vi "TDT-AODO-Engine.vi"(0 "Config":T1, 2 "Action":T3, 5 "AO":dbl[][](array[numeric]), 7 "DO":bool[][](array[boolean]), 11 "error in (no error)":errorcluster) -> (6 "next buffer":i32, 8 "Space Available":dbl, 15 "error out":errorcluster)   [LabVIEW 2020]
uses:
  Typedefs/TDT-AODO-Action.ctl
  Typedefs/TDT-AODO-Config.ctl
  Typedefs/TDT-AODO-Output Spec.ctl
  TDT-Globals.vi
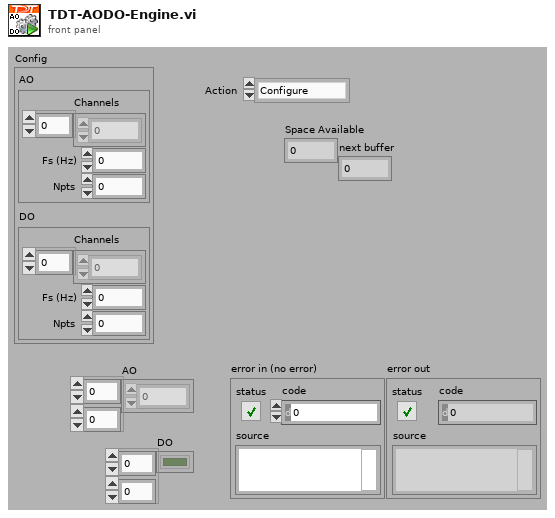
[diagram p1: front panel]
types:
  T1 = typedef "TDT-AODO-Config.ctl" = cluster{"AO":T2, "DO":T2}
  T2 = typedef "TDT-AODO-Output Spec.ctl" = cluster{"Channels":i32[], "Fs (Hz)":dbl, "Npts":i32}
  T3 = typedef "TDT-AODO-Action.ctl" = enum16{"Configure", "Initialize", "Start", "Stop", "Write", "Clean up", "Space available"}
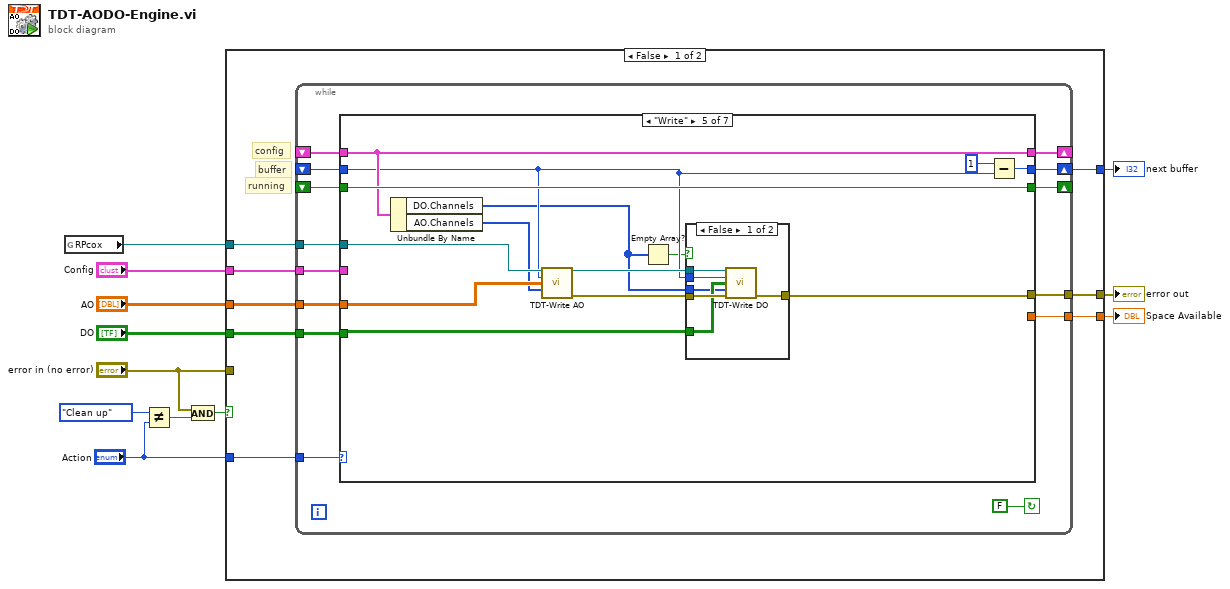
[diagram p0: block diagram]
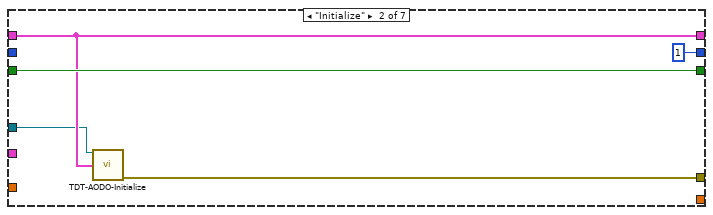
[diagram p3: hidden frame]
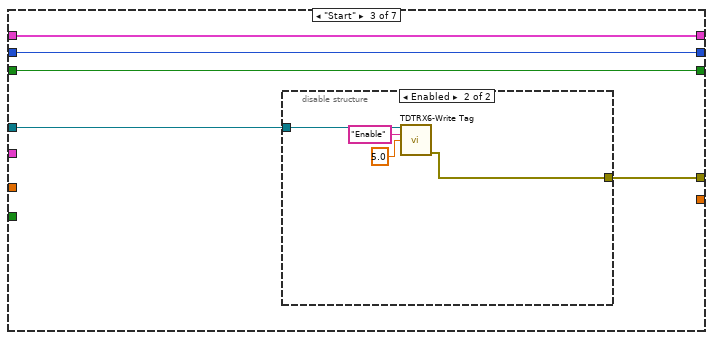
[diagram p4: hidden frame]
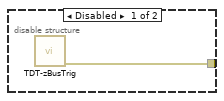
[diagram p5: hidden frame]
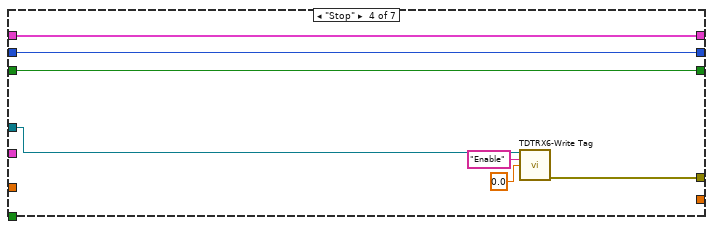
[diagram p6: hidden frame]
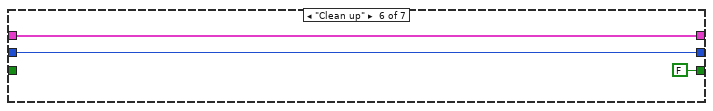
[diagram p8: hidden frame]
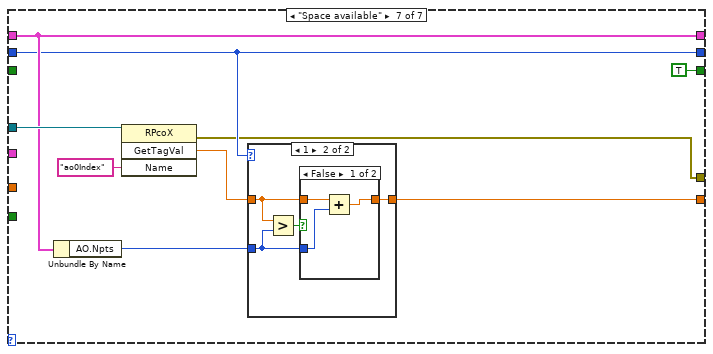
[diagram p9: hidden frame]
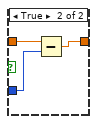
[diagram p11: hidden frame]
diagram:
  n1 = global read "TDT-Globals.vi" "RPcox"() -> (w2:refnum<k7>)
  n2 = Not Equal?(x=TDT-AODO-Action."Clean up", y="Action") -> (x != y?=w6:bool)
  n3 = And(x="error in (no error)", y=w6) -> (x .and. y?=w7:bool)
  n4 = case shown="False" w7 {
    tunnel: "Action" -> [w20 _]
    tunnel: [w19 w104] -> w12
    tunnel: "Config" -> [w18 _]
    tunnel: "AO" -> [w17 _]
    tunnel: "error in (no error)" -> [_ w104]
    tunnel: "DO" -> [w16 _]
    tunnel: [w15 _] -> w3
    tunnel: w2 -> [w14 _]
    tunnel: [w13 _] -> w1
    frame False {
      # "running"
      # "config"
      # "buffer"
      n5 = while {
        shift-right: [w28] -> w13
        shift-left: _ -> [w33]
        tunnel: [w32] -> w19
        tunnel: w18 -> [w30]
        shift-right: [w31] -> _
        shift-left: _ -> [w29]
        tunnel: w17 -> [w27]
        tunnel: w16 -> [w26]
        tunnel: w20 -> [w34]
        tunnel: [w24] -> w15
        shift-right: [w23] -> _
        shift-left: _ -> [w22]
        tunnel: w14 -> [w21]
        stop <- FALSE continue-if-true
        n6 = case shown="\"Write\"" w34 {
          tunnel: [_ w41 w44 w54 w71 _ w84] -> w32
          tunnel: w33 -> [w36 _ w46 w58 w62 w83 w88]
          tunnel: [w37 w40 w47 w59 w68 w82 w90] -> w31
          tunnel: w30 -> [w37 _ _ _ _ _ _]
          tunnel: w29 -> [_ w40 w47 w59 w68 w82 w90]
          tunnel: [w36 1 w46 w58 w64 w83 w88] -> w28
          tunnel: w27 -> [_ _ _ _ w69 _ _]
          tunnel: w26 -> [_ _ _ _ w73 _ _]
          tunnel: [_ _ _ _ _ _ w87] -> w24
          tunnel: [w35 w42 w45 w57 w72 FALSE TRUE] -> w23
          tunnel: w22 -> [w35 w42 w45 w57 w72 _ _]
          tunnel: w21 -> [_ w39 w43 w53 w70 _ w91]
          frame "Configure", Default {
          }
          frame "Initialize" {
            n7 = call "TDT-AODO-Initialize.vi"("RPcox"=w39, "Config"=w40) -> ("error out"=w41:errorcluster)  [unwired: 13 in]
          }
          frame "Start" {
            n8 = disable-structure shown="Enabled" {
              disable-tunnel: [w48 w49] -> w44
              disable-tunnel: w43 -> [_ w52]
              frame Disabled {
                n9 = call "TDT-zBusTrig.vi"() -> ("error out"=w48:errorcluster)  [unwired: 7 in]
              }
              frame Enabled {
                n10 = call "TDTRX6-Write Tag.vi"("RPcox"=w52, "Name"="Enable", "Value"=sgl 5.0) -> ("error out"=w49:errorcluster)  [unwired: 11 in, 1 out]
              }
            }
          }
          frame "Stop" {
            n11 = call "TDTRX6-Write Tag.vi"("RPcox"=w53, "Name"="Enable", "Value"=sgl 0.0) -> ("error out"=w54:errorcluster)  [unwired: 11 in, 1 out]
          }
          frame "Write" {
            n12 = Unbundle By Name(w68) -> ("DO.Channels"=w60:i32[], "AO.Channels"=w67:i32[])
            n13 = call "TDT-Write AO.vi"("RPcox"=w70, "Next Buffer"=w62, "Input array"=w69, "Chans"=w67) -> ("RPcox (thru)"=w65:refnum<k7>, "error out"=w66:errorcluster)  [unwired: 10 in]
            n14 = Empty Array?(array=w60) -> (empty?=w61:bool)
            n15 = case shown="False" w61 {
              tunnel: w66 -> [w79 w80]
              tunnel: w73 -> [w76 _]
              tunnel: [w78 w80] -> w71
              tunnel: w65 -> [w77 _]
              tunnel: w62 -> [w75 _]
              tunnel: w60 -> [w74 _]
              frame False {
                n16 = call "TDT-Write DO.vi"("RPcox"=w77, "Next Buffer"=w75, "Input array"=w76, "Chans"=w74, "error in (no error)"=w79) -> ("error out"=w78:errorcluster)  [unwired: 9 in, 1 out]
              }
              frame True {
              }
            }
            n17 = Subtract(x=1, y=w62) -> (x-y=w64:i32)
          }
          frame "Clean up" {
          }
          frame "Space available" {
            n18 = Unbundle By Name(w90) -> ("AO.Npts"=w86:i32)
            n19 = invoke class="RPcoX" method="GetTagVal"(reference=w91, "Name"="ao0Index") -> (error out=w84:errorcluster, "GetTagVal"=w85:sgl)  [unwired: 2 in, 2 out]
            n20 = case shown="1" w88 {
              tunnel: w85 -> [w93 w96]
              tunnel: [w93 w94] -> w87
              tunnel: w86 -> [_ w95]
              frame 0, Default {
              }
              frame 1 {
                n21 = Greater?(x=w96, y=w95) -> (0:w97:bool)
                n22 = case shown="False" w97 {
                  tunnel: w96 -> [w100 w102]
                  tunnel: w95 -> [w99 w101]
                  tunnel: [w98 w103] -> w94
                  frame False {
                    n23 = Add(x=w100, y=w99) -> (x+y=w98:sgl)
                  }
                  frame True {
                    n24 = Subtract(x=w102, y=w101) -> (x-y=w103:sgl)
                  }
                }
              }
            }
          }
        }
      }
    }
    frame True {
    }
  }
  "error out" <- w12
  "Space Available" <- w3
  "next buffer" <- w1
